vi "uniformRandom.vi"(7 "samples":u32, 10 "lower":u32, 11 "upper":u32) -> (3 "randnum":u32[](array[numeric]))   [LabVIEW 2019]
uses:
  <vilib>/Analysis/NI_AALBase.lvlib
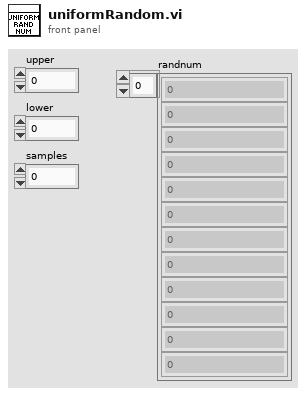
[diagram p1: front panel]
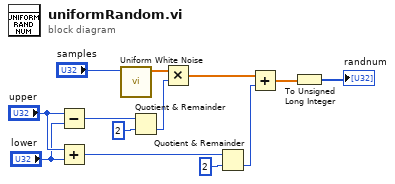
[diagram p0: block diagram]
diagram:
  n1 = Subtract(x="upper", y="lower") -> (x-y=w12:u32)
  n2 = Add(x="upper", y="lower") -> (x+y=w8:u32)
  n3 = call <vilib>:"Uniform White Noise.vi"("samples"="samples") -> ("uniform white noise"=w5:dbl[])  [unwired: 9 in, 1 out]
  n4 = Quotient & Remainder(x=w12, y=u32 2) -> (floor(x/y)=w4:u32)  [unwired: 1 out]
  n5 = Multiply(x=w5, y=w4) -> (x*y=w3:dbl[])
  n6 = Quotient & Remainder(x=w8, y=u32 2) -> (floor(x/y)=w6:u32)  [unwired: 1 out]
  n7 = Add(x=w3, y=w6) -> (x+y=w2:dbl[])
  n8 = To Unsigned Long Integer(number=w2) -> (unsigned 32bit integer=→"randnum":u32[])
